vi "Track Goal.vi"(7 "Original Image":T3(plugin-control), 9 "Camera Type":T4, 10 "Targets":T5(array[cluster]), 11 "Goal Display":T3(plugin-control)) -> (1 "Target Line Masking Out":T3(plugin-control), 2 "Best Target Available":T2, 3 "Found Targets":T6(array[cluster]) {"Normalized Rect"."Numeric 5" format="%#_2g"; "Normalized Rect"."Numeric 3" format="%#_2g"; "Normalized Rect"."Numeric 2" format="%#_2g"; "Normalized Rect"."Numeric" format="%#_2g"}, 5 "Goal Display":T3(plugin-control))   [LabVIEW 2015]
uses:
  Camera Types.ctl
panel:
  out "Sorted Scores":T1(array[cluster]) {"Moment Factor" format="%#_3g"; "L" format="%#_3g"; "Area to CH" format="%#_3g"; "X" format="%#_3g"; "Y" format="%#_3g"}
  # "Aspect Ratio"
  # "Density Profile"
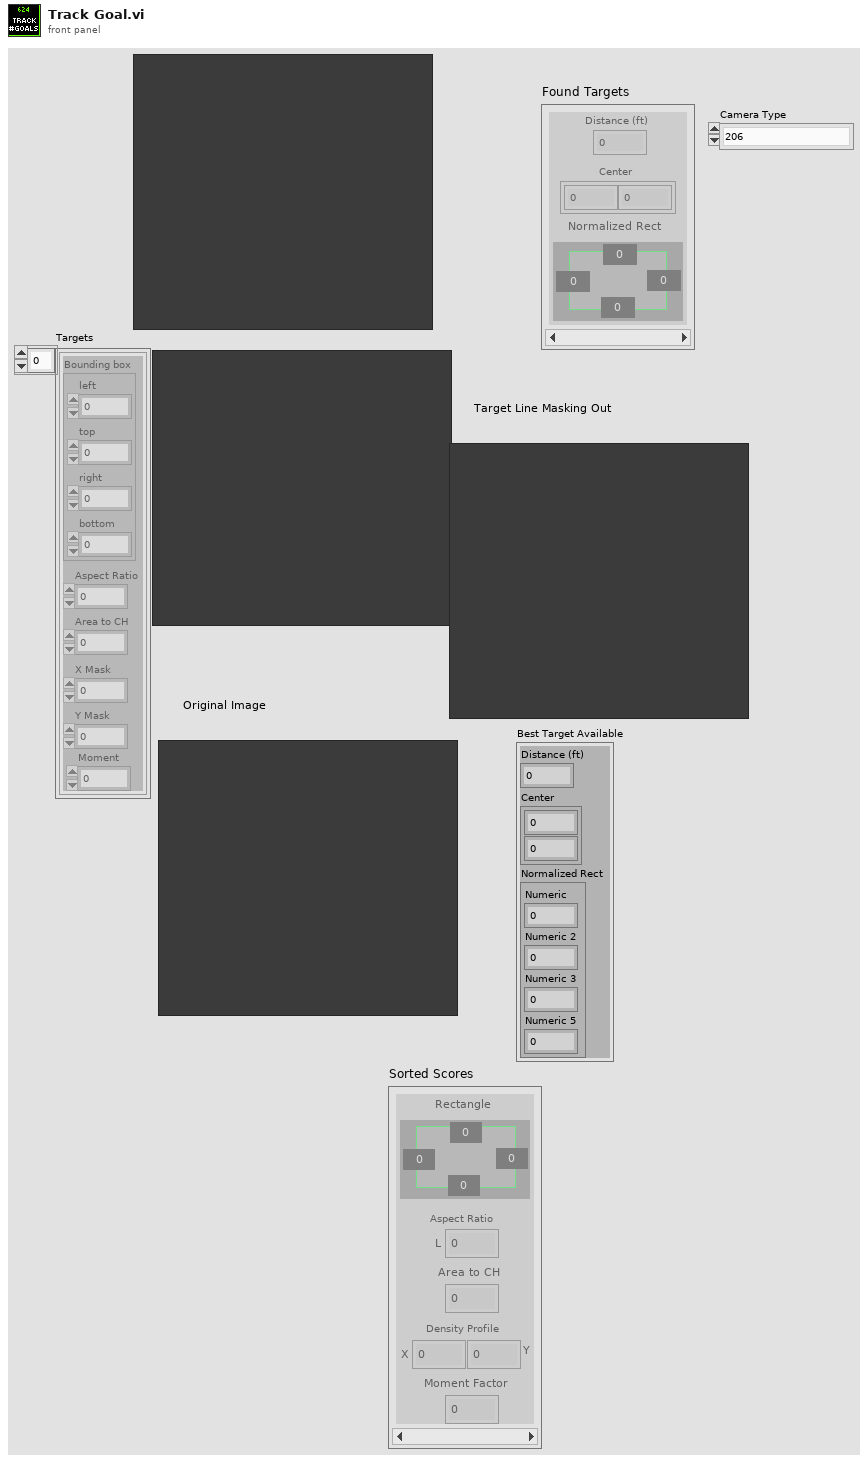
[diagram p1: front panel]
types:
  T1 = cluster{"Rectangle":cluster{"Numeric":dbl, "Numeric 2":dbl, "Numeric 3":dbl, "Numeric 5":dbl}, "L":dbl, "Area to CH":dbl, "X":dbl, "Y":dbl, "Moment Factor":dbl}[]
  T2 = cluster{"Distance (ft)":dbl, "Center":cluster{dbl, dbl}, "Normalized Rect":cluster{"Numeric":dbl, "Numeric 2":dbl, "Numeric 3":dbl, "Numeric 5":dbl}}
  T3 = typedef "IMAQ Image.ctl" = refnum<image>
  T4 = typedef "Camera Types.ctl" = enum16{"206", "1011", "1013", "MS HD3000 square", "MS HD3000 640x480"}
  T5 = cluster{"Bounding box":cluster{"left":dbl, "top":dbl, "right":dbl, "bottom":dbl}, "Aspect Ratio":dbl, "Area to CH":dbl, "X Mask":dbl, "Y Mask":dbl, "Moment":dbl}[]
  T6 = cluster{"Distance (ft)":dbl, "Center":cluster{dbl, dbl}, "Normalized Rect":cluster{"Numeric":dbl, "Numeric 2":dbl, "Numeric 3":dbl, "Numeric 5":dbl}}[]
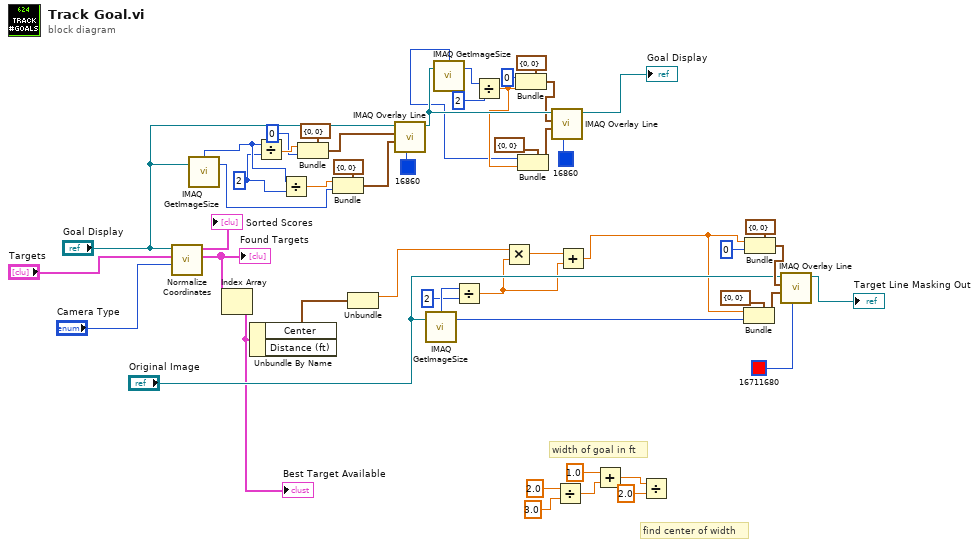
[diagram p0: block diagram]
diagram:
  w40 = 2 ("y")
  # "find center of width"
  # "width of goal in ft"
  n1 = call "Normalize Coordinates.vi"("Camera Type"="Camera Type", "Targets"="Targets", "Image in"="Goal Display") -> ("Found Targets"=w17:T6, "Sorted Scores"=→"Sorted Scores":T1)  [unwired: 7 in]
  "Found Targets" <- w17
  n2 = call "IMAQ GetImageSize"("Image"="Goal Display") -> ("Y Resolution"=w38:i32, "X Resolution"=w41:i32)  [unwired: 3 in, 1 out]
  n3 = Index Array(array=w17) -> (element=w16:T2)  [unwired: 1 in]
  "Best Target Available" <- w16
  n4 = Unbundle By Name(w16) -> ("Center"=w15:cluster{dbl, dbl})  [unwired: 1 out]
  n5 = Divide(x=w41, y=w40) -> (x/y=w46:dbl)
  n6 = Divide(x=w41, y=w40) -> (x/y=w44:dbl)
  n7 = Bundle(cluster=cluster{"X":i32, "Y":i32} {"X"=0, "Y"=0} ("Start Point"), "X"=w46, "Y"=0) -> (w42:cluster{"X":i32, "Y":i32})
  n8 = Bundle(cluster=cluster{"X":i32, "Y":i32} {"X"=0, "Y"=0} ("Start Point"), "X"=w44, "Y"=w38) -> (w39:cluster{"X":i32, "Y":i32})
  n9 = Unbundle(w15) -> (w11:dbl)  [unwired: 1 out]
  n10 = call "IMAQ Overlay Line"("Color"=u32 16860, "End Point"=w39, "Start Point"=w42, "Image"="Goal Display") -> ("Image Out"=w37:T3)  [unwired: 6 in, 1 out]
  n11 = call "IMAQ GetImageSize"("Image"="Original Image") -> ("Y Resolution"=w18:i32, "X Resolution"=w13:i32)  [unwired: 3 in, 1 out]
  n12 = call "IMAQ GetImageSize"("Image"=w37) -> ("Y Resolution"=w35:i32, "X Resolution"=w28:i32)  [unwired: 3 in, 1 out]
  n13 = Divide(x=w13, y=2) -> (x/y=w9:dbl)
  n14 = Divide(x=w35, y=2) -> (x/y=w29:dbl)
  n15 = Multiply(x=w11, y=w9) -> (x*y=w10:dbl)
  n16 = Bundle(cluster=cluster{"X":i32, "Y":i32} {"X"=0, "Y"=0} ("Start Point"), "X"=0, "Y"=w29) -> (w30:cluster{"X":i32, "Y":i32})
  n17 = Bundle(cluster=cluster{"X":i32, "Y":i32} {"X"=0, "Y"=0} ("Start Point"), "X"=w28, "Y"=w29) -> (w27:cluster{"X":i32, "Y":i32})
  n18 = call "IMAQ Overlay Line"("Color"=u32 16860, "End Point"=w27, "Start Point"=w30, "Image"=w37) -> ("Image Out"=→"Goal Display":T3)  [unwired: 6 in, 1 out]
  n19 = Divide(x=2.0, y=3.0) -> (x/y=w4:dbl)
  n20 = Add(x=w10, y=w9) -> (x+y=w8:dbl)
  n21 = Add(x=1.0, y=w4) -> (x+y=w2:dbl)
  n22 = Divide(x=w2, y=2.0) -> ()  [unwired: 1 out]
  n23 = Bundle(cluster=cluster{"X":i32, "Y":i32} {"X"=0, "Y"=0} ("Start Point"), "X"=w8, "Y"=w18) -> (w24:cluster{"X":i32, "Y":i32})
  n24 = Bundle(cluster=cluster{"X":i32, "Y":i32} {"X"=0, "Y"=0} ("Start Point"), "X"=w8, "Y"=0 ("X")) -> (w23:cluster{"X":i32, "Y":i32})
  n25 = call "IMAQ Overlay Line"("Color"=u32 16711680, "End Point"=w24, "Start Point"=w23, "Image"="Original Image") -> ("Image Out"=→"Target Line Masking Out":T3)  [unwired: 6 in, 1 out]
